vi "ROI_crop.vi"(8 "error constant":errorcluster, 10 "roiEdge":T1, 11 "InputImage":dbl[][](array[numeric])) -> (0 "error constant 2":errorcluster, 3 "ROI":dbl[][](array[numeric]))   [LabVIEW 2014]
doc: "This SubVI is used to crop the ROIs out of the input images."
uses:
  TypeDef/ROIedge.ctl
panel:
  # "This SubVI is used to crop the ROIs out of the input images."
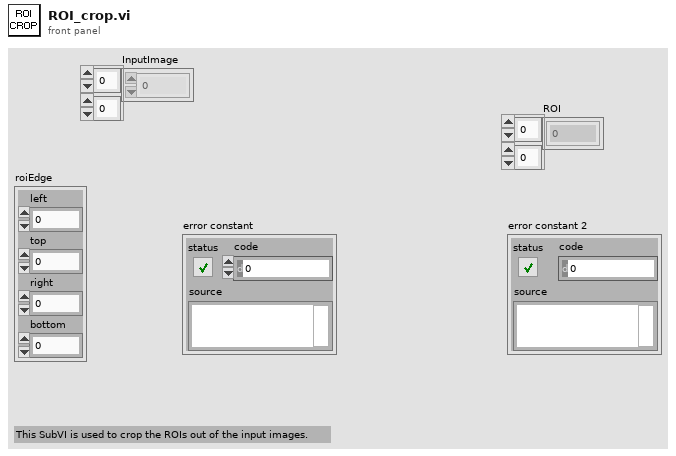
[diagram p1: front panel]
types:
  T1 = typedef "ROIedge.ctl" = cluster{"left":i16, "top":i16, "right":i16, "bottom":i16}
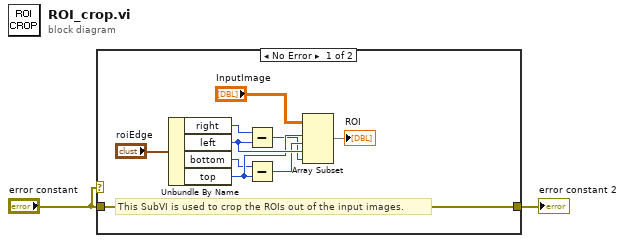
[diagram p0: block diagram]
diagram:
  n1 = case shown="No Error" "error constant" {
    tunnel: "error constant" -> [w5 w13]
    tunnel: [w5 w13] -> w1
    frame No Error {
      # "This SubVI is used to crop the ROIs out of the input images."
      n2 = Unbundle By Name("roiEdge") -> ("right"=w6:i16, "left"=w12:i16, "bottom"=w7:i16, "top"=w11:i16)
      n3 = Subtract(x=w6, y=w12) -> (x-y=w9:i16)
      n4 = Subtract(x=w7, y=w11) -> (x-y=w10:i16)
      n5 = Array Subset(array="InputImage", index (row)=w11, length (row)=w10, index (col)=w12, length (col)=w9) -> (→"ROI":dbl[][])
    }
    frame Error {
    }
  }
  "error constant 2" <- w1
